vi "read diff arg settings.vi"(8 "error in (no error)":errorcluster, 10 "VIscc Path":path=path "C:/viscc") -> (0 "error out":errorcluster, 1 "UseDefault?":bool, 2 "ActiveDiffArgs":T1)   [LabVIEW 2016]
uses:
  ActiveDiffArgs.ctl
  <vilib>/Utility/config.llb/Read Key (Boolean).vi
  <vilib>/Utility/config.llb/Write Key (Boolean).vi
  <vilib>/Utility/config.llb/NI_LVConfig.lvlib
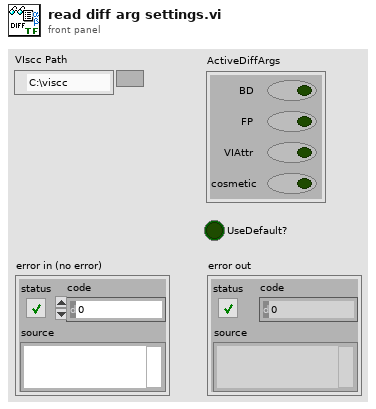
[diagram p1: front panel]
types:
  T1 = typedef "ActiveDiffArgs.ctl" = cluster{"BD":bool, "FP":bool, "VIAttr":bool, "cosmetic":bool}
  T2 = typedef "NI_LVConfig.lvlib/Config Data RefNum.ctl" = refnum<k1>
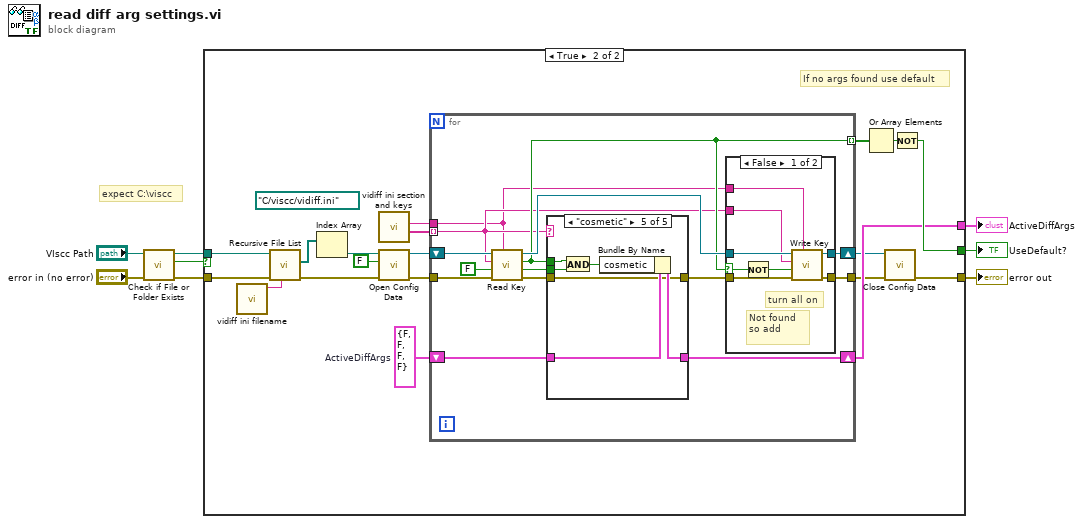
[diagram p0: block diagram]
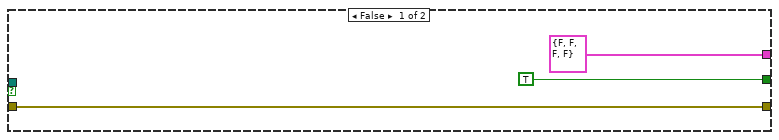
[diagram p2: hidden frame]
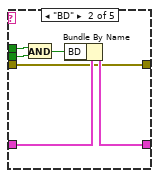
[diagram p5: hidden frame]
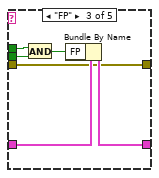
[diagram p6: hidden frame]
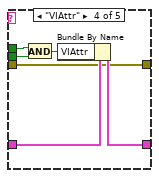
[diagram p7: hidden frame]
diagram:
  # "expect C:\\viscc"
  n1 = call <vilib>:"Check if File or Folder Exists.vi"("error in (no error)"="error in (no error)", "path"="VIscc Path") -> ("error out"=w3:errorcluster, "file or folder exists?"=w2:bool, "dup path"=w5:path)  [unwired: 7 in]
  n2 = case shown="True" w2 {
    tunnel: [w10 w13] -> w8
    tunnel: w5 -> [_ w29]
    tunnel: [TRUE w16] -> w7
    tunnel: w3 -> [w10 w28]
    tunnel: [T1 {"BD"=FALSE, "FP"=FALSE, "VIAttr"=FALSE, "cosmetic"=FALSE} ("ActiveDiffArgs") w15] -> w1
    frame False {
    }
    frame True {
      w19 = T1 {"BD"=FALSE, "FP"=FALSE, "VIAttr"=FALSE, "cosmetic"=FALSE}  # ActiveDiffArgs
      (unwired) path "C:/viscc/vidiff.ini" ("VIscc Path")
      # "If no args found use default"
      n3 = call "vidiff ini filename.vi"() -> ("VIdiff INI file"=w27:string)  [unwired: 11 in]
      n4 = call <vilib>:"Recursive File List.vi"("pattern"=w27, "error in (no error)"=w28, "Folder Path"=w29) -> ("error out"=w25:errorcluster, "All Files in Dir"=w30:path[])  [unwired: 4 in, 3 out]
      n5 = Index Array(array=w30) -> (element=w26:path)  [unwired: 1 in]
      n6 = call "vidiff ini section and keys.vi"() -> ("DiffArgKeyNames"=w20:string[], "Section"=w22:string)  [unwired: 10 in]
      n7 = call <vilib>:"Open Config Data.vi"("error in (no error)"=w25, "create file if necessary (T)"=FALSE, "configuration file path"=w26) -> ("error out"=w21:errorcluster, "refnum"=w23:T2)  [unwired: 6 in, 1 out]
      n8 = for {
        tunnel: w22 -> [w31]
        tunnel: w21 -> [w43]
        tunnel: w20 -> [w32] mode=indexing
        tunnel: [w35] -> w14
        shift-right: [w37] -> w12
        shift-left: w23 -> [w44]
        shift-right: [w39] -> w15
        shift-left: w19 -> [w40]
        tunnel: [w33] -> w18 mode=indexing
        n9 = call-poly <vilib>:"Read Key.vi"("section"=w31, "error in (no error)"=w43, "default value"=FALSE, "key"=w32, "refnum"=w44) -> ("error out"=w38:errorcluster, "value"=w41:bool, "found?"=w33:bool, "refnum out"=w34:T2)  [unwired: 3 in]
        n10 = case shown="\"cosmetic\"" w32 {
          tunnel: w33 -> [_ w60 w66 w72 w78]
          tunnel: w41 -> [_ w61 w67 w73 w79]
          tunnel: w40 -> [w55 w62 w68 w74 w80]
          tunnel: [w55 w59 w65 w71 w77] -> w39
          tunnel: w38 -> [w56 w57 w63 w69 w75]
          tunnel: [w56 w57 w63 w69 w75] -> w36
          frame Default {
          }
          frame "BD" {
            n11 = And(x=w60, y=w61) -> (x .and. y?=w58:bool)
            n12 = Bundle By Name(cluster=w62, "BD"=w58) -> (w59:T1)
          }
          frame "FP" {
            n13 = And(x=w66, y=w67) -> (x .and. y?=w64:bool)
            n14 = Bundle By Name(cluster=w68, "FP"=w64) -> (w65:T1)
          }
          frame "VIAttr" {
            n15 = And(x=w72, y=w73) -> (x .and. y?=w70:bool)
            n16 = Bundle By Name(cluster=w74, "VIAttr"=w70) -> (w71:T1)
          }
          frame "cosmetic" {
            n17 = And(x=w78, y=w79) -> (x .and. y?=w76:bool)
            n18 = Bundle By Name(cluster=w80, "cosmetic"=w76) -> (w77:T1)
          }
        }
        n19 = case shown="False" w33 {
          selector: w33 -> [w47 _]
          tunnel: [w52 w54] -> w37
          tunnel: w36 -> [w51 w53]
          tunnel: [w50 w53] -> w35
          tunnel: w34 -> [w49 w54]
          tunnel: w32 -> [w48 _]
          tunnel: w31 -> [w45 _]
          frame False {
            # "turn all on"
            # "Not found\nso add"
            n20 = Not(x=w47) -> (.not. x?=w46:bool)
            n21 = call-poly <vilib>:"Write Key.vi"("section"=w45, "error in (no error)"=w51, "value"=w46, "key"=w48, "refnum"=w49) -> ("error out"=w50:errorcluster, "refnum out"=w52:T2)  [unwired: 4 in, 1 out]
          }
          frame True {
          }
        }
      }
      n22 = Or Array Elements(Boolean array=w18) -> (logical OR=w17:bool)
      n23 = call <vilib>:"Close Config Data.vi"("error in (no error)"=w14, "refnum"=w12) -> ("error out"=w13:errorcluster)  [unwired: 8 in, 1 out]
      n24 = Not(x=w17) -> (.not. x?=w16:bool)
    }
  }
  "error out" <- w8
  "UseDefault?" <- w7
  "ActiveDiffArgs" <- w1
